vi "PH_OceanOpticsSpectrometer.set Trigger Info.vi"(0 "i ref in":refnum<vi>, 5 "error in (no error)":errorcluster) -> (14 "i ref out":refnum<vi>, 19 "error out":errorcluster)   [LabVIEW 2014, in "PH_OceanOpticsSpectrometer.lvlib"]
doc: "This VI sets GUI information in case of external triggering."
uses:
  PH_OceanOpticsSpectrometer.lvlib
  PH_Common/PH_Common.lvlib
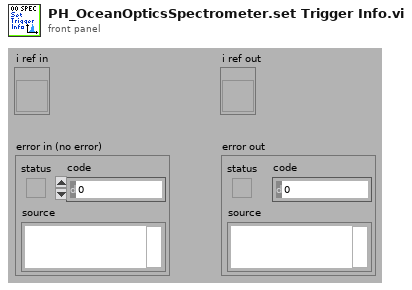
[diagram p1: front panel]
types:
  T1 = typedef "PH_OceanOpticsSpectrometer.lvlib/PH_OceanOpticsSpectrometer.i attribute.ctl" = cluster{"GUI Refs":cluster{"Delete":refnum<vi>, "Spectrum":refnum<vi>, "Display Width":refnum<vi>, "Display Center":refnum<vi>, "Save":refnum<vi>, "Integration time":refnum<vi>, "center wavelength":refnum<vi>, "width":refnum<vi>, "Wanted Trigger Mode":refnum<vi>, "Current Trigger Mode":refnum<vi>, "Trigger Info":refnum<vi>, "Model":refnum<vi>, "Driver":refnum<vi>, "Firmware":refnum<vi>}, "Display":cluster{"Width":dbl, "Center":dbl}, "VISA resource name":refnum<visa-resource-name>, "Integration time [ms]":cluster{"Current Value":u16, "Wanted Value":u16}, "Trigger":cluster{"Current value":T2, "Wanted value":T2}, "Default VISA Timeout":u32, "Last Data":cluster{"Wavelength Bins":dbl[], "Spectrum by Pixels":dbl[]}}
  T2 = typedef "PH_OceanOpticsSpectrometer.lvlib/PH_OceanOpticsSpectrometer.Trigger.ctl" = enum32{"External", "Normal"}
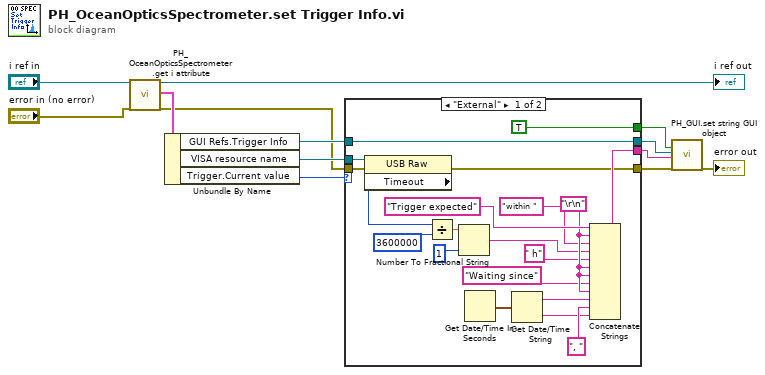
[diagram p0: block diagram]
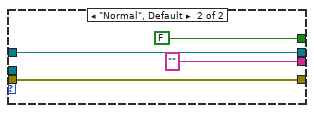
[diagram p2: hidden frame]
diagram:
  n1 = call "PH_OceanOpticsSpectrometer.get i attribute.vi"("i ref in"="i ref in", "error in (no error)"="error in (no error)") -> ("i ref out"=→"i ref out":refnum<vi>, "i attribute"=w13:T1, "error out"=w1:errorcluster)  [unwired: 15 in]
  n2 = Unbundle By Name(w13) -> ("GUI Refs.Trigger Info"=w9:refnum<vi>, "VISA resource name"=w7:refnum<visa-resource-name>, "Trigger.Current value"=w8:T2)
  n3 = case shown="\"External\"" w8 {
    tunnel: [w22 ""] -> w6
    tunnel: w7 -> [w21 _]
    tunnel: [TRUE FALSE] -> w5
    tunnel: w1 -> [w18 w34]
    tunnel: [w17 w35] -> w4
    tunnel: w9 -> [w17 w35]
    tunnel: [w16 w34] -> w3
    frame "External" {
      w32 = "\r\n"
      n4 = property class="USB Raw"(reference=w21, error in=w18) -> (error out=w16:errorcluster, "Timeout"=w20:u32)  [unwired: 1 out]
      n5 = Divide(x=w20, y=u32 3600000 ("Default VISA Timeout")) -> (x/y=w29:dbl)
      n6 = Number To Fractional String(number=w29, precision (6)=i16 1 ("width (-)")) -> (F-format string=w31:string)  [unwired: 2 in]
      n7 = Get Date/Time In Seconds() -> (seconds since 1Jan1904=w23:timestamp)
      n8 = Get Date/Time String(seconds (now)=w23) -> (date string=w25:string, time string=w26:string)  [unwired: 2 in]
      n9 = Concatenate Strings("Trigger expected", w32, "within ", w31, " h", w32, w32, "Waiting since" ("string"), w32, w25, ", " ("string"), w26) -> (w22:string)
    }
    frame "Normal", Default {
    }
  }
  n10 = call "PH_GUI.set string GUI object.vi"("Visible (True)"=w5, "GUI object Ref"=w4, "Text"=w6, "error in"=w3) -> ("error out"=→"error out":errorcluster)  [unwired: 15 in]
